vi "MainPC.vi"() -> ()   [LabVIEW 2018]
uses:
  <vilib>/Platform/TimedLoop/XDataNode/timing_clust.ctl
  <vilib>/Platform/TimedLoop/XDataNode/nitl_modes.ctl
  <vilib>/Platform/TimedLoop/XDataNode/wakeup.ctl
  <vilib>/platform/TimedLoop/XDataNode/XDataNode.xnode
  <vilib>/Platform/TimedLoop/XDataNode/XDNodeRunTimeDep.lvlib
panel:
  in  "Stop Motor":bool
  in  "Disconnect":bool
  in  "Frequency [Hz]":dbl(knob)=1000.0 scale=0.0..10000.0
  in  "Duty Cycle":dbl(slide)=0.5 scale=0.0..1.0
  out "Status":bool
  in  "Quit":bool
  # "Overview: \nGUI on PC controlling Foucault Pendulum on myRIO\nInstructions:\nStart/Disconnect to connect/disconnect to/from myRIO\nStop to quit both Apps."
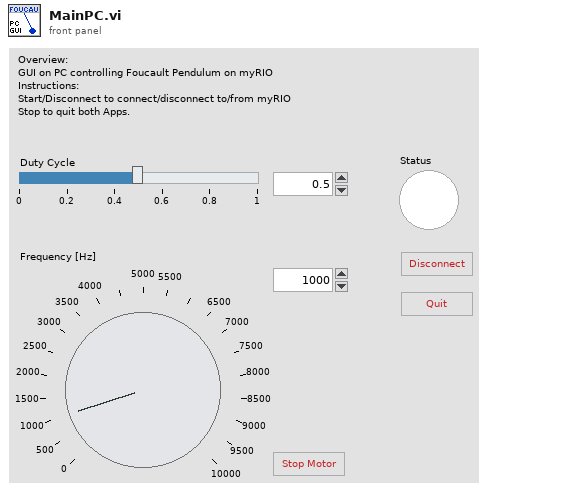
[diagram p1: front panel]
types:
  T1 = typedef "XDNodeRunTimeDep.lvlib/timing_clust.ctl" = cluster{"Expected End [f-1]":u64, "Actual End [f-1]":u64, "Finished Late? [f-1]":bool, "Expected End [i-1]":u64, "Actual End [i-1]":u64, "Finished Late? [i-1]":bool, "Expected Start [i]":u64, "Actual Start [i]":u64, "Expected Start [f]":u64, "Actual Start [f]":u64, "Source Name":string, "Structure Name":string, "Period":i64, "Deadline":i64, "Offset":i64, "Start":i64, "Priority":i32, "Timeout":i32, "Mode":T2, "Wakeup Reason":T3, "Error":errorcluster, "Source Type":string, "Secondary Source Type":string, "Global End Time":u64, "Global Start Time":u64, "Frame Duration":u64, "Iteration Duration":u64, "Assigned CPU":i32, "I/O Scan Engine Mode":u32}
  T2 = typedef "XDNodeRunTimeDep.lvlib/nitl_modes.ctl" = enum32{"No Change", "Process missed periods, maintain original phase", "Discard missed periods, maintain original phase", "Process missed periods, ignore original phase", "Discard missed periods, ignore original phase"}
  T3 = typedef "XDNodeRunTimeDep.lvlib/wakeup.ctl" = enum32{"Normal", "Aborted", "Asynchronous wakeup", "Timing source error", "Timed loop error", "Timeout"}
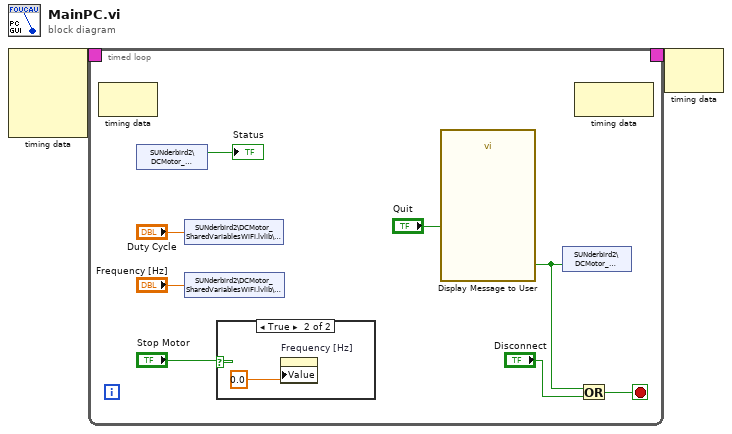
[diagram p0: block diagram]
diagram:
  n1 = node-c288() -> (w2:T1)  [unwired: 4 in]
  n2 = timed-loop {
    timing: w2 -> [_]
    timing-out: [_] -> w1
    stop <- w7 stop-if-true
    n3 = node-c288() -> ()  [unwired: 1 in, 1 out]
    n4 = shared-variable "SUNderbird2\\DCMotor_SharedVariablesWiFi.lvlib\\LED0"() -> (→"Status":bool)  [unwired: 1 in, 1 out]
    n5 = shared-variable "SUNderbird2\\DCMotor_SharedVariablesWiFi.lvlib\\DutyCycle"("Duty Cycle") -> ()  [unwired: 1 in, 1 out]
    n6 = shared-variable "SUNderbird2\\DCMotor_SharedVariablesWiFi.lvlib\\Frequency"("Frequency [Hz]") -> ()  [unwired: 1 in, 1 out]
    n7 = case shown="True" "Stop Motor" {
      frame False {
      }
      frame True {
        n8 = property on="Frequency [Hz]" class="Knob (strict)"("Value"=0.0 ("Frequency [Hz]")) -> ()  [unwired: 2 in, 2 out]
      }
    }
    n9 = call "Display Message to User"("Enable"="Quit") -> ("Ja"=w3:bool)  [unwired: 9 in, 1 out]
    n10 = shared-variable "SUNderbird2\\DCMotor_SharedVariablesWiFi.lvlib\\Stop"(w3) -> ()  [unwired: 1 in, 1 out]
    n11 = node-c288() -> ()  [unwired: 1 in, 1 out]
    n12 = Or(x=w3, y="Disconnect") -> (x .or. y?=w7:bool)
  }
  n13 = node-c288(w1) -> ()  [unwired: 1 out]
